vi "AnalogAlicat.vi"() -> ()   [LabVIEW 2018]
uses:
  <vilib>/DAQmx/read.llb/DAQmx Read (Analog 1D Wfm NChan NSamp).vi
  <vilib>/DAQmx/write.llb/DAQmx Write (Analog DBL 1Chan 1Samp).vi
  <vilib>/DAQmx/configure/timing.llb/DAQmx Timing (Sample Clock).vi
  <vilib>/DAQmx/configure/task.llb/DAQmx Configure Logging (TDMS).vi
  <vilib>/DAQmx/miscellaneous.llb/DAQmx Fill In Error Info.vi
  <resource>/objmgr/daqmx.rc
panel:
  in  "Flush Rate":u32=100 min=1 step=1
  in  "Reset":bool
  out "XY Graph":cluster{"Y":dbl[], "Y":dbl[]}[](graph)=[{"Y"=[3646920262.9766912, 3646920263.076691, 3646920263.176691, 3646920263.2766914, 3646920263.3766913, 3646920263.4766912, 3646920263.576691, 3646920263.676691, 3646920263.7766914, 3646920263.8766913, 3646920263.9766912, 3646920264.076691, 3646920264.176691, 3646920264.3096914, 3646920264.4236913, 3646920264.523691, 3646920264.623691, 3646920264.723691, 3646920264.8236914, 3646920264.9236913, 3646920265.023691, 3646920265.123691, 3646920265.223691, 3646920265.3446913, 3646920265.4806914, 3646920265.5806913, 3646920265.6806912, 3646920265.779691, 3646920265.879691, 3646920265.979691, 3646920266.0796914, 3646920266.189691, 3646920266.322691, 3646920266.4226913, 3646920266.5226912, 3646920266.656691, 3646920266.756691, 3646920266.8566914, 3646920266.9566913, 3646920267.056691, 3646920267.156691, 3646920267.3646913, 3646920267.5266914, 3646920267.6266913, 3646920267.7266912, 3646920267.826691, 3646920267.926691, 3646920268.0266914, 3646920268.1266913, 3646920268.2266912, 3646920268.359691, 3646920268.459691, 3646920268.5596914, 3646920268.6596913, 3646920268.759691, 3646920268.859691, 3646920268.959691, 3646920269.0596914, 3646920269.1596913, 3646920269.289691, 3646920269.3896914, 3646920269.4896913, 3646920269.589691, 3646920269.689691, 3646920269.789691, 3646920269.8896914, 3646920269.9896913, 3646920270.089691, 3646920270.189691, 3646920270.314691, 3646920270.414691, 3646920270.5146914, 3646920270.6146913, 3646920270.714691, 3646920270.814691, 3646920270.914691, 3646920271.0146914, 3646920271.1146913, 3646920271.214691, 3646920271.333691, 3646920271.433691, 3646920271.5336914, 3646920271.6336913, 3646920271.733691, 3646920271.833691, 3646920271.933691, 3646920272.0336914, 3646920272.1336913, 3646920272.233691, 3646920272.367691, 3646920272.4676914, 3646920272.5676913, 3646920272.667691, 3646920272.767691, 3646920272.867691, 3646920272.9676914, 3646920273.0676913, 3646920273.167691, 3646920273.2976913, 3646920273.3976912, 3646920273.497691, 3646920273.597691, 3646920273.697691, 3646920273.7976913, 3646920273.8976912, 3646920273.997691, 3646920274.097691, 3646920274.197691, 3646920274.321691, 3646920274.440691, 3646920274.5406914], "Y"=[-0.014524225021772353, 0.02264186807147099, -0.018908573932329545, -0.055490100454245524, 0.010528159720130765, -0.0035796684146618364, 0.03385277450577464, 0.16197910038812616, -0.04603295272954757, -0.07824963907369771, 0.12873611558990267, 0.022862707262761094, 0.15772010329665104, 0.11010533346024037, 0.06777017381074243, 0.09629209201293384, 0.08666604751767332, 0.19010373207905862, 0.1472282690787513, 0.037626556043905905, 0.058632352662868516, -0.09258476468352372, 0.13012483667760746, 0.11565439926838281, -0.07813920941058124, 0.05057166794981174, -0.04380984263896997, 0.12271502110171773, 0.2886764621711312, 0.035541536743813225, 0.15331181139665423, 0.2885256658062023, 0.1066585997695948, 0.21303215401509878, 0.08557862685275029, 0.10085829620766129, 0.1572375112519469, 0.09240789963842928, 0.0034352579515365377, -0.06573319568134636, 0.06171198780610999, 0.10928486499474231, -0.05791285973208405, 0.06864161322461465, -0.06051098321675864, -0.15209472102963562, 0.10931517759007409, 0.06601750855017602, 0.14983935437776008, 0.17447700160664195, 0.18192840642074942, 0.10472950285774647, 0.1493327288708962, 0.1293402074938194, 0.3377029632615669, 0.18387474224346012, 0.09365969058099073, -0.0016733103525773544, 0.15066327510310165, 0.06912888330053166, 0.05233636361331568, -0.05043675928608215, 0.05172600487862405, 0.06430221618682544, 0.008170338558573334, -0.08757038913463575, -0.09474119991715683, 0.03209902590576764, 0.10980036543871073, 0.349563400767982, 0.17124788604326455, -0.08749245932683233, 0.17843167014333042, -0.01822657092728011, 0.19547534667345964, 0.13720601117928147, -0.07730132198692752, -0.021006554524455164, 0.04908425425666315, 0.02877342577260684, 0.26462432942653813, 0.08995268427446856, 0.07522134212456652, -0.10109362733638821, 0.004149771379108211, -0.08097765630346222, 0.036626265899784516, 0.08873156139290168, 0.09727017529677454, -0.03723181220513282, 0.008183348179362018, 0.005851521724238676, 0.01669218883767163, 0.14035621770612094, 0.12925576344064996, -0.07259873183627476, 0.019654035162166458, 0.06839277478914126, -0.04205782214476436, -0.11164847757784672, 0.01923833481184144, 0.1341921719706369, 0.06765431274065263, 0.07622812747830637, -0.234097904484781, 0.18595324523015788, 0.011859685770773868, 0.08839339014723624, -0.26196196801865684, 0.15352869252368395]}]
  out "Arithmetic Mean":dbl=0.15352869252368395
  in  "Flow Rate [CCM]":dbl format="%0.2f"
  in  "Analog Out":refnum<k21>="MyVoltageOutTask_0"
  in  "Set Flow":bool
  in  "samples per channel":i32=100
  in  "rate":dbl=1000.0 format="%0.2f"
  in  "Analog In":refnum<k21>="MyVoltageTask"
  in  "stop":bool
  in  "Wait time[ms]":u32=100
  out "File Size (Mb)":dbl=0.029935836791992188
  out "output cluster":cluster{"data":waveform(dbl)[]}
  out "Filepath":path=path "H:/Data/Raw Data/2019-07-25/Logfiles/MyVoltageTask/RawDAQmx/Log_MyVoltageTask_1_DAQmx.tdms"
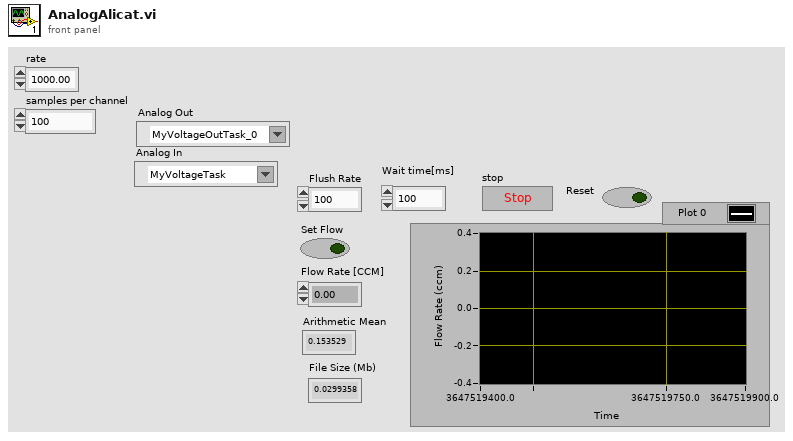
[diagram p1: front panel]
types:
  T1 = enum16{"open", "open or create", "create or replace", "create", "open (read-only)"}
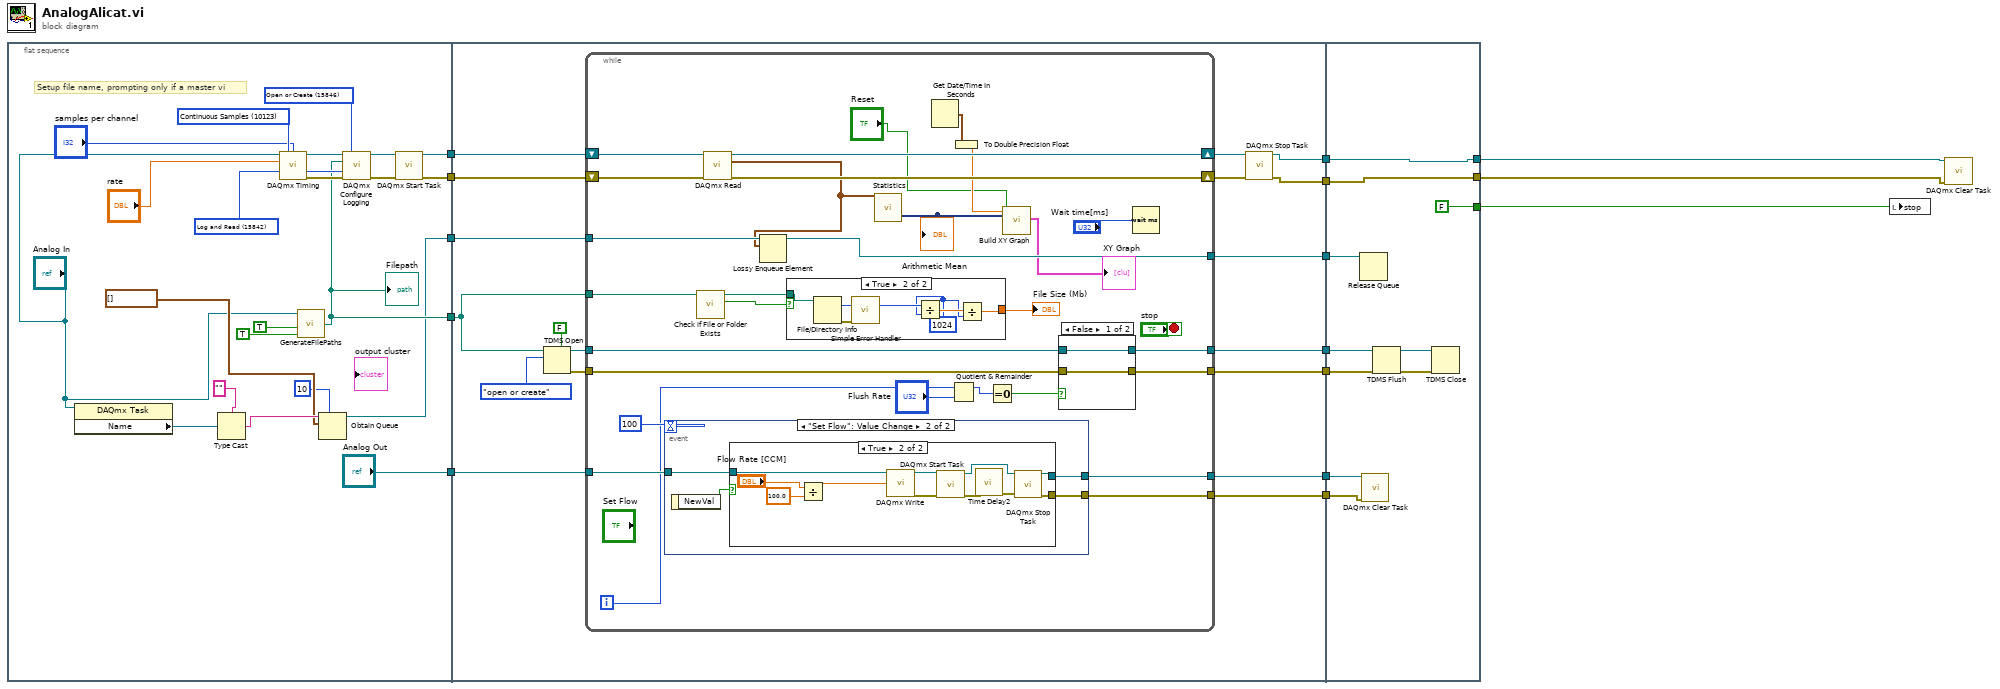
[diagram p0: block diagram]
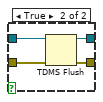
[diagram p2: hidden frame]
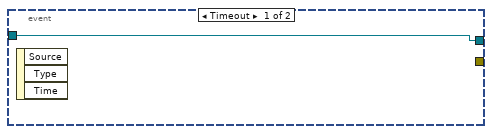
[diagram p3: hidden frame]
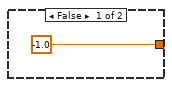
[diagram p5: hidden frame]
diagram:
  n1 = flat-sequence {
    tunnel: [w36] -> w15
    tunnel: [w37] -> w14
    tunnel: [w26] -> w11
    tunnel: [w22] -> w10
    tunnel: ["Analog Out"] -> w1
    tunnel: w15 -> [w55]
    tunnel: w14 -> [w54]
    tunnel: [w53] -> w13
    tunnel: [w52] -> w12
    tunnel: w11 -> [w47]
    tunnel: w10 -> [w45]
    tunnel: [w44] -> w9
    tunnel: [w43] -> w7
    tunnel: [w42] -> w6
    tunnel: [w40] -> w3
    tunnel: [w39] -> w2
    tunnel: w1 -> [w38]
    tunnel: w13 -> [w123]
    tunnel: w12 -> [w125]
    tunnel: w9 -> [w121]
    tunnel: [FALSE ("stop")] -> w8
    tunnel: w7 -> [w119]
    tunnel: w6 -> [w118]
    tunnel: [w119] -> w5
    tunnel: [w118] -> w4
    tunnel: w3 -> [w117]
    tunnel: w2 -> [w116]
    frame #0 {
      w27 = 10123 items=["Finite Samples"=10178, "Continuous Samples"=10123, "Hardware Timed Single Point"=12522] ("sample mode")
      w28 = 15846 items=["Open"=10437, "Open or Create"=15846, "Create or Replace"=15847, "Create"=15848] ("operation")
      w29 = 15842 items=["Off"=10231, "Log"=15844, "Log and Read"=15842] ("logging mode")
      # "Setup file name, prompting only if a master vi"
      n2 = property class="DAQmx Task"(reference="Analog In") -> ("Name"=w25:refnum<k21>)  [unwired: 1 in, 2 out]
      n3 = Type Cast(type="", x=w25) -> (*(type *) &x=w23:string)
      n4 = call-poly <vilib>:"DAQmx Timing.vi"("task/channels in"="Analog In", "sample mode"=w27, "samples per channel"="samples per channel", "rate"="rate") -> ("task out"=w31:refnum<k21>, "error out"=w30:errorcluster)  [unwired: 10 in]
      n5 = call "GenerateFilePaths.vi"("Logfile? (F)"=TRUE ("Instrument? (create folder)"), "DAQmx (F)"=TRUE ("DAQmx"), "Device Name"="Analog In") -> ("Path"=w26:path)  [unwired: 1 in]
      "Filepath" <- w26
      n6 = Obtain Queue(max queue size (-1, unlimited)=10, name (unnamed)=w23, element data type=waveform(dbl)[] [] ("data")) -> (queue out=w22:refnum<queue>)  [unwired: 2 in, 2 out]
      n7 = call-poly <vilib>:"DAQmx Configure Logging.vi"("task/channels in"=w31, "operation"=w28, "file path"=w26, "logging mode"=w29, "error in"=w30) -> ("task out"=w33:refnum<k21>, "error out"=w32:errorcluster)  [unwired: 9 in]
      n8 = call <vilib>:"DAQmx Start Task.vi"("task/channels in"=w33, "error in"=w32) -> ("task out"=w36:refnum<k21>, "error out"=w37:errorcluster)  [unwired: 12 in]
    }
    frame #1 {
      n9 = TDMS Open(5:FALSE ("create index file? (T)"), 10:T1."open or create" ("operation (0:open)"), 11:w47) -> (0:w49:errorcluster, 3:w48:refnum<k34>)  [unwired: 4 in]
      n10 = while {
        shift-right: [w85] -> w46
        shift-left: w54 -> [w81]
        shift-right: [w82] -> w41
        shift-left: w55 -> [w83]
        tunnel: w48 -> [w77]
        tunnel: w49 -> [w76]
        tunnel: [w79] -> w52
        tunnel: [w78] -> w53
        tunnel: w47 -> [w72]
        tunnel: w45 -> [w71]
        tunnel: [w69] -> w44
        tunnel: [w67] -> w40
        tunnel: [w66] -> w39
        tunnel: w38 -> [w65]
        i -> [w59]
        stop <- "stop" stop-if-true
        n11 = event shown="[1] \"Set Flow\": Value Change" {
          selector: _ -> [_ _]
          dyn-events: _ -> [_ _]
          timeout: 100 -> [_ _]
          tunnel: [w92 w96] -> w67
          tunnel: [_ w95] -> w66
          tunnel: w65 -> [w92 w94]
          event Timeout {
            n12 = event-data() -> ()  [unwired: 1 in, 3 out]
          }
          event "Set Flow": Value Change {
            n13 = event-data() -> ("NewVal"=w93:bool)  [unwired: 1 in]
            n14 = case shown="True" w93 {
              tunnel: [w97 w103] -> w96
              tunnel: [_ w102] -> w95
              tunnel: w94 -> [w97 w101]
              frame False {
              }
              frame True {
                n15 = Divide(x="Flow Rate [CCM]", y=100.0) -> (x/y=w100:dbl)
                n16 = call-poly <vilib>:"DAQmx Write.vi"("task/channels in"=w101, "data"=w100) -> ("task out"=w108:refnum<k21>, "error out"=w107:errorcluster)  [unwired: 11 in, 1 out]
                n17 = call <vilib>:"DAQmx Start Task.vi"("task/channels in"=w108, "error in"=w107) -> ("task out"=w104:refnum<k21>, "error out"=w106:errorcluster)  [unwired: 12 in]
                n18 = call "Time Delay2"("error in (no error)"=w106) -> ("error out"=w105:errorcluster)  [unwired: 10 in]
                n19 = call <vilib>:"DAQmx Stop Task.vi"("task/channels in"=w104, "error in"=w105) -> ("task out"=w103:refnum<k21>, "error out"=w102:errorcluster)  [unwired: 12 in]
              }
            }
          }
        }
        n20 = call <vilib>:"Check if File or Folder Exists.vi"("path"=w72) -> ("file or folder exists?"=w74:bool, "dup path"=w75:path)  [unwired: 8 in, 1 out]
        n21 = call-poly <vilib>:"DAQmx Read.vi"("task/channels in"=w83, "error in"=w81) -> ("task out"=w82:refnum<k21>, "data"=w70:waveform(dbl)[], "error out"=w85:errorcluster)  [unwired: 11 in]
        n22 = Lossy Enqueue Element(queue=w71, element=w70) -> (queue out=w69:refnum<queue>)  [unwired: 1 in, 3 out]
        n23 = case shown="True" w74 {
          tunnel: [-1.0 w110] -> w73
          tunnel: w75 -> [_ w113]
          frame False {
          }
          frame True {
            w111 = i64 1024 ("y")
            n24 = File/Directory Info(path=w113) -> (size=w115:i64, error out=w114:errorcluster)  [unwired: 1 in, 5 out]
            n25 = call <vilib>:"Simple Error Handler.vi"("error in (no error)"=w114) -> ()  [unwired: 1 in, 8 out]
            n26 = Divide(x=w115, y=w111) -> (x/y=w112:dbl)
            n27 = Divide(x=w112, y=w111) -> (x/y=w110:dbl)
          }
        }
        "File Size (Mb)" <- w73
        n28 = call "Statistics"("Signals"=w70) -> ("Arithmetic Mean"=w63:dynamicdata)  [unwired: 25 in, 1 out]
        "Arithmetic Mean" <- w63
        n29 = Get Date/Time In Seconds() -> (seconds since 1Jan1904=w62:timestamp)
        n30 = Quotient & Remainder(x=w59, y="Flush Rate") -> (x-y*floor(x/y)=w57:u32)  [unwired: 1 out]
        n31 = To Double Precision Float(number=w62) -> (double precision float=w61:dbl)
        n32 = Equal To 0?(x=w57) -> (x = 0?=w56:bool)
        n33 = call "Build XY Graph"("Reset"="Reset", "Y Input"=w63, "X Input"=w61) -> ("XY Graph"=→"XY Graph":cluster{"X":dbl[], "Y":dbl[]}[])  [unwired: 7 in, 1 out]
        n34 = case shown="False" w56 {
          tunnel: [w87 w91] -> w79
          tunnel: [w86 w90] -> w78
          tunnel: w77 -> [w87 w89]
          tunnel: w76 -> [w86 w88]
          frame False {
          }
          frame True {
            n35 = TDMS Flush(4:w88, 7:w89) -> (0:w90:errorcluster, 3:w91:refnum<k34>)
          }
        }
        n36 = Wait (ms)(milliseconds to wait="Wait time[ms]") -> ()  [unwired: 1 out]
      }
      n37 = call <vilib>:"DAQmx Stop Task.vi"("task/channels in"=w41, "error in"=w46) -> ("task out"=w43:refnum<k21>, "error out"=w42:errorcluster)  [unwired: 12 in]
    }
    frame #2 {
      n38 = Release Queue(queue=w121) -> ()  [unwired: 2 in, 3 out]
      n39 = call <vilib>:"DAQmx Clear Task.vi"("task in"=w117, "error in"=w116) -> ()  [unwired: 13 in, 1 out]
      n40 = TDMS Flush(4:w123, 7:w125) -> (0:w122:errorcluster, 3:w124:refnum<k34>)
      n41 = TDMS Close(8:w122, 11:w124) -> ()  [unwired: 2 out]
    }
  }
  n42 = local write "stop"(w8) -> ()
  n43 = call <vilib>:"DAQmx Clear Task.vi"("task in"=w5, "error in"=w4) -> ()  [unwired: 13 in, 1 out]
